vi "I2C Write Byte.vi"(8 "error in (no error)":errorcluster, 9 "Value":u8, 10 "Register Address":u8, 11 "LINX I2C in":refnum<class "LINX I2C.lvclass">) -> (0 "error out":errorcluster, 3 "LINX I2C out":refnum<class "LINX I2C.lvclass">)   [LabVIEW 2020, in "LINX I2C.lvclass"]
doc: "Writes bytes to the I2C bus."
uses:
  LINX I2C.lvclass
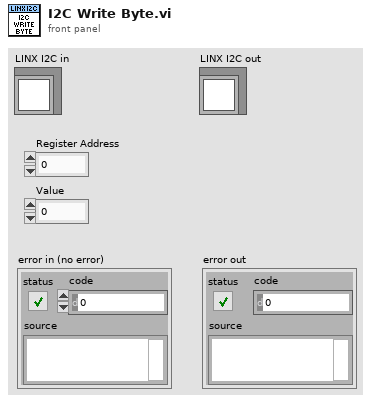
[diagram p1: front panel]
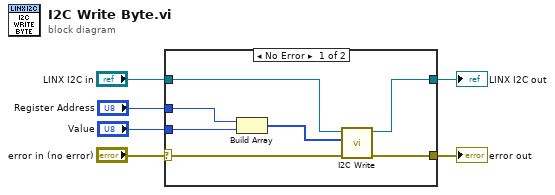
[diagram p0: block diagram]
diagram:
  n1 = case shown="No Error" "error in (no error)" {
    selector: "error in (no error)" -> [w13 w14]
    tunnel: [w10 w15] -> w6
    tunnel: "LINX I2C in" -> [w12 w15]
    tunnel: [w11 w14] -> w4
    tunnel: "Register Address" -> [w9 _]
    tunnel: "Value" -> [w8 _]
    frame No Error {
      n2 = Build Array(w9, w8) -> (w7:u8[])
      n3 = call "I2C Write.vi"("error in (no error)"=w13, "Bytes to Write"=w7, "LINX I2C in"=w12) -> ("error out"=w11:errorcluster, "LINX I2C out"=w10:refnum<class "LINX I2C.lvclass">)  [unwired: 7 in]
    }
    frame Error {
    }
  }
  "LINX I2C out" <- w6
  "error out" <- w4
